vi "Create Plot Object.vi"(6 "Control Ref Queue":T1, 7 "Actual Transform In":T2, 8 "error in (no error)":errorcluster, 9 "Multiplot Representation In":T4, 10 "3D Bar.lvclass in":refnum<class "3D Bar.lvclass">, 11 "Plot Object In":refnum<vi>) -> (0 "error out":errorcluster, 1 "Multiplot Representation Out":T4, 2 "3D Bar.lvclass out":refnum<class "3D Bar.lvclass">, 3 "Plot Object Out":refnum<vi>, 5 "Actual Transform Out":T2)   [LabVIEW 2017, in "3D Bar.lvclass"]
uses:
  <vilib>/Math Plots/3D Math Plots/3D Bar/3D Bar/3D Bar.lvclass
  <vilib>/Math Plots/3D Math Plots/3D Plot/3D Plot/Typedef/Multiplot Representation.ctl
  <vilib>/Math Plots/3D Math Plots/3D Plot/3D Plot/Typedef/Plot Representation.ctl
  <vilib>/Math Plots/3D Math Plots/3D Plot/3D Plot/Typedef/Range Clusters.ctl
  <vilib>/Math Plots/3D Math Plots/3D Plot/3D Plot/Typedef/Mesh Data.ctl
  <vilib>/Math Plots/3D Math Plots/3D Plot/3D Plot/Typedef/Actual Transform.ctl
  <vilib>/Math Plots/3D Math Plots/3D Plot/Action String/3DMathPlot Ctrl Act Queue.ctl
  <vilib>/Math Plots/3D Math Plots/3D Plot/Action String/3DMathPlot Ctrl Act Cluster.ctl
  <vilib>/Math Plots/3D Math Plots/3D Plot/Action String/3DMathPlot State Class.ctl
  <vilib>/Math Plots/3D Math Plots/3D Bar/3D Bar/3D Bar.lvclass/3D Bar.ctl
  <vilib>/Math Plots/3D Math Plots/3D Plot/3D Plot/3D Plot.lvclass
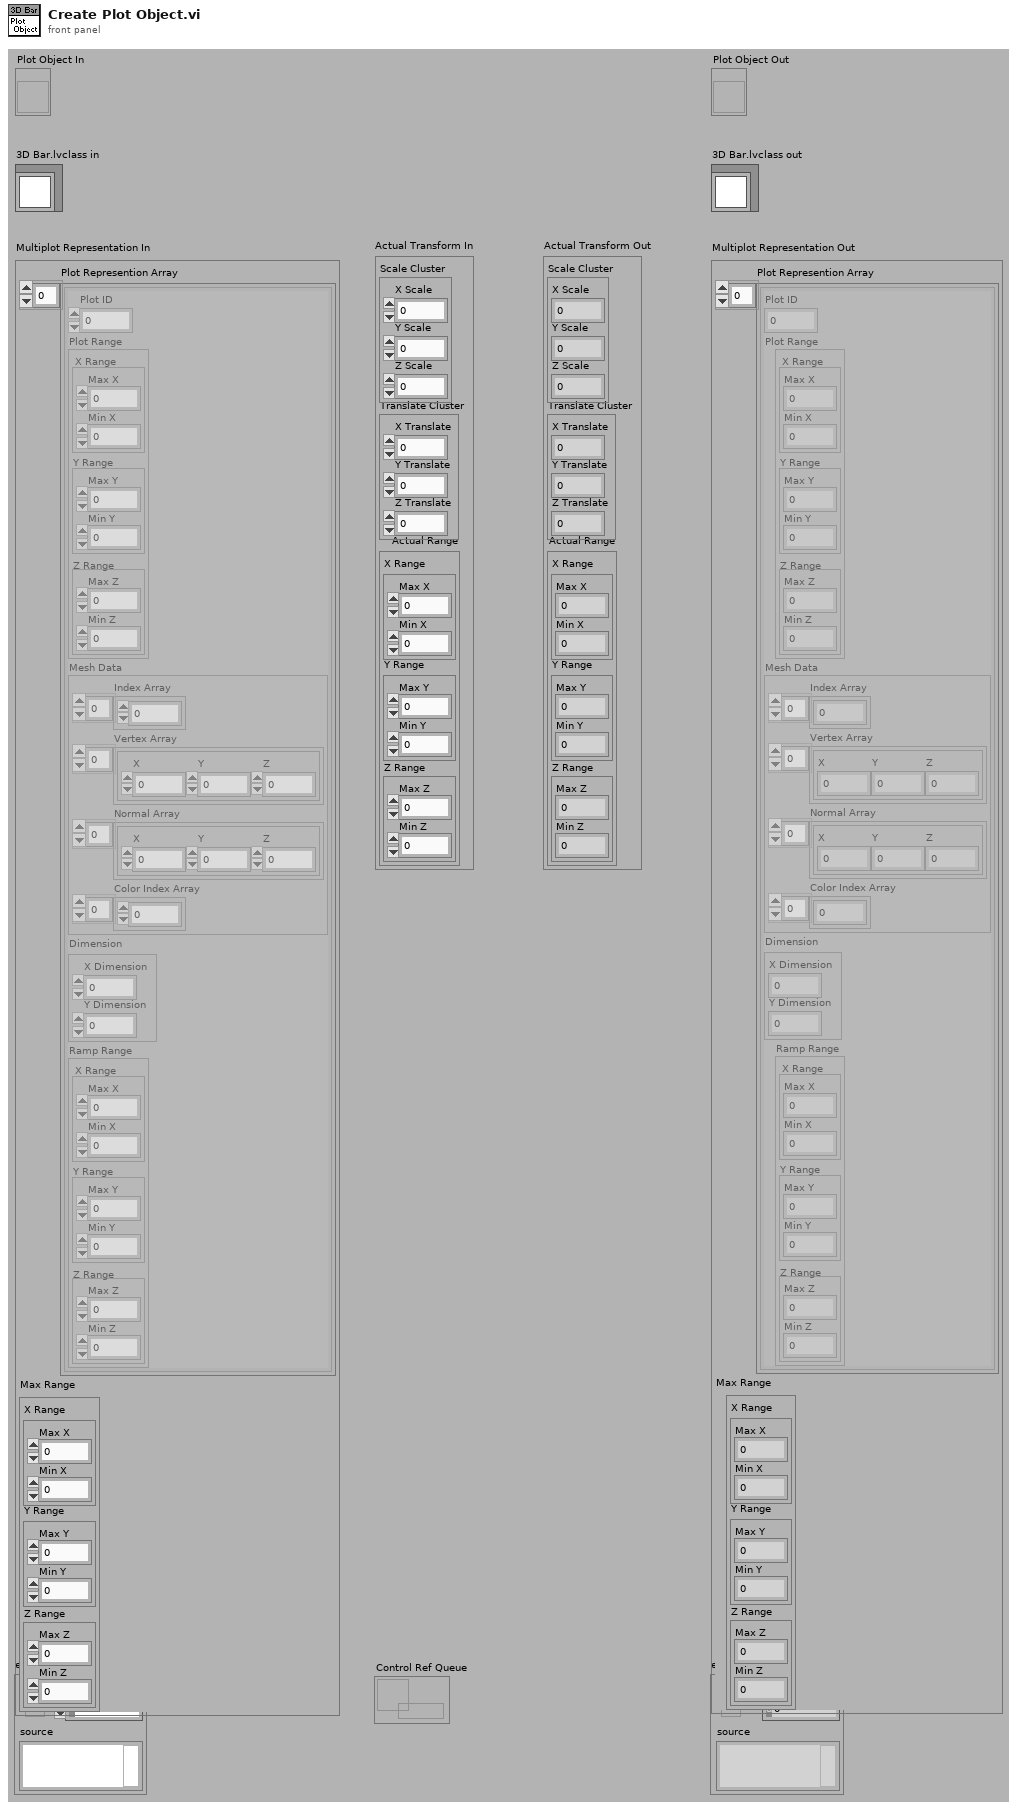
[diagram p1: front panel]
types:
  T1 = typedef "3DMathPlot Ctrl Act Queue.ctl" = refnum<queue>
  T2 = typedef "3D Plot.lvclass/Actual Transform.ctl" = cluster{"Scale Cluster":cluster{"X Scale":sgl, "Y Scale":sgl, "Z Scale":sgl}, "Translate Cluster":cluster{"X Translate":sgl, "Y Translate":sgl, "Z Translate":sgl}, "Actual Range":T3}
  T3 = typedef "3D Plot.lvclass/Range Clusters.ctl" = cluster{"X Range":cluster{"Max X":sgl, "Min X":sgl}, "Y Range":cluster{"Max Y":sgl, "Min Y":sgl}, "Z Range":cluster{"Max Z":sgl, "Min Z":sgl}}
  T4 = typedef "3D Plot.lvclass/Multiplot Representation.ctl" = cluster{"Plot Represention Array":T5[], "Max Range":T3}
  T5 = typedef "3D Plot.lvclass/Plot Representation.ctl" = cluster{"Plot ID":i32, "Plot Range":T3, "Mesh Data":T6, "Dimension":cluster{"X Dimension":i32, "Y Dimension":i32}, "Ramp Range":T3}
  T6 = typedef "3D Plot.lvclass/Mesh Data.ctl" = cluster{"Index Array":u32[], "Vertex Array":cluster{"X":sgl, "Y":sgl, "Z":sgl}[], "Normal Array":cluster{"X":sgl, "Y":sgl, "Z":sgl}[], "Color Index Array":i32[]}
  T7 = typedef "3D Bar.lvclass/3D Bar Property Array.ctl" = T8[]
  T8 = typedef "3D Bar.lvclass/3D Bar Property.ctl" = cluster{"General Property":cluster{"Plot Name":string, "Coordinate System":enum16{"Cartesian", "Cylindrical", "Spherical"}, "Opacity":sgl}, "Projection Property":cluster{"Draw XY":bool, "Draw YZ":bool, "Draw XZ":bool}, "Plot Property":cluster{"Line Style":T9, "Line Width":sgl, "Line Color":u32, "Antialiasing":bool}, "Bar Property":cluster{"Bar Mode":enum16{"Detach", "Group", "Stack"}, "Bar Width":sgl, "Color Pair Array":cluster{"Color":u32, "String":string}[]}}
  T9 = typedef "3D Plot.lvclass/Line Type.ctl" = enum16{"None", "Solid", "Dash", "Dot", "Dash Dot"}
  T10 = enum16{"Points", "Lines", "Line Strip", "Line Loop", "Triangles", "Triangle Strip", "Triangle Fan", "Quads", "Quad Strip", "Polygon"}
  T11 = cluster{"Draw XY":bool, "Draw YZ":bool, "Draw XZ":bool}
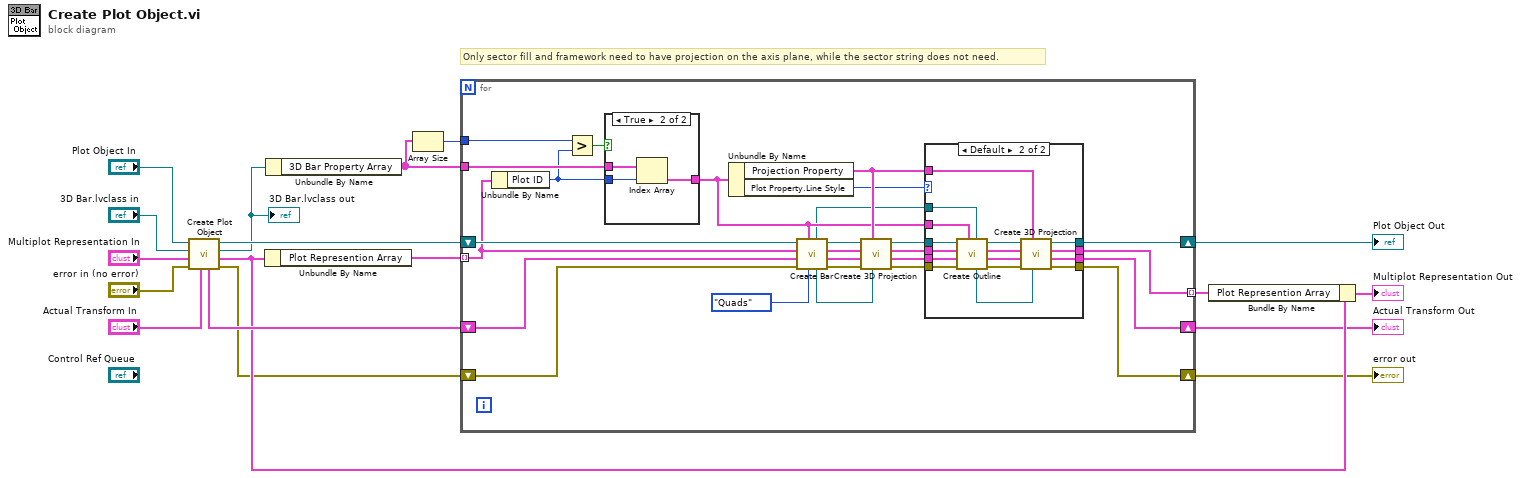
[diagram p0: block diagram]
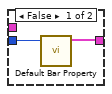
[diagram p2: hidden frame]
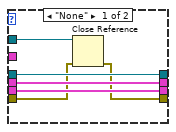
[diagram p3: hidden frame]
diagram:
  # "Only sector fill and framework need to have projection on the axis plane, while the sector string does not need."
  n1 = call-parent "Create Plot Object.vi"("Actual Transform In"="Actual Transform In", "error in (no error)"="error in (no error)", "Multiplot Representation In"="Multiplot Representation In", "3D Plot.lvclass in"="3D Bar.lvclass in", "Plot Object In"="Plot Object In") -> ("error out"=w3:errorcluster, "Multiplot Representation Out"=w10:T4, "3D Plot.lvclass out"=w4:refnum<class "3D Bar.lvclass">, "Plot Object Out"=w6:refnum<vi>, "Actual Transform Out"=w11:T2)  [unwired: 1 in, 1 out]
  "3D Bar.lvclass out" <- w4
  n2 = Unbundle By Name(w10) -> ("Plot Represention Array"=w18:T5[])
  n3 = Unbundle By Name(w4) -> ("3D Bar Property Array"=w1:T7)
  n4 = Array Size(array=w1) -> (size(s)=w2:i32)
  n5 = for {
    tunnel: [w38] -> w17 mode=indexing
    shift-right: [w37] -> w5
    shift-left: w6 -> [w41]
    shift-right: [w39] -> w7
    shift-left: w3 -> [w40]
    shift-right: [w36] -> w8
    shift-left: w11 -> [w42]
    tunnel: w18 -> [w28] mode=indexing
    tunnel: w1 -> [w25]
    tunnel: w2 -> [w22]
    n6 = Unbundle By Name(w28) -> ("Plot ID"=w24:i32)
    n7 = Greater?(x=w22, y=w24) -> (0:w26:bool)
    n8 = case shown="True" w26 {
      tunnel: w25 -> [_ w47]
      tunnel: [w43 w46] -> w23
      tunnel: w24 -> [w44 w45]
      frame False {
        n9 = call <vilib>:"Default Bar Property.vi"("Plot ID"=w44) -> ("Default Property"=w43:T8)  [unwired: 10 out]
      }
      frame True {
        n10 = Index Array(array=w47, index=w45) -> (element=w46:T8)
      }
    }
    n11 = Unbundle By Name(w23) -> ("Projection Property"=w29:T11, "Plot Property.Line Style"=w27:T9)
    n12 = call <vilib>:"Create Bar.vi"("Draw Mode"=T10."Quads", "3D Bar Property"=w23, "error in (no error)"=w40, "Plot Representation In"=w28, "Plot Object In"=w41) -> ("error out"=w35:errorcluster, "Plot Representation Out"=w32:T5, "Plot Object Out"=w34:refnum<vi>, "Sector Object Out"=w20:refnum<vi>, "Bar Drawable"=w19:refnum<vi>)  [unwired: 2 out]
    n13 = call <vilib>:"Create 3D Projection.vi"("Sub Object In"=w20, "Projection Property"=w29, "error in (no error)"=w35, "Actual Transform In"=w42, "Plot Object In"=w34) -> ("error out"=w33:errorcluster, "Actual Transform Out"=w30:T2, "Plot Object Out"=w31:refnum<vi>)  [unwired: 1 in, 3 out]
    n14 = case shown="Default" w27 {
      tunnel: [w48 w67] -> w39
      tunnel: [w52 w66] -> w38
      tunnel: [w53 w65] -> w37
      tunnel: [w51 w64] -> w36
      tunnel: w33 -> [w49 w63]
      tunnel: w32 -> [w52 w62]
      tunnel: w31 -> [w53 w61]
      tunnel: w30 -> [w51 w60]
      tunnel: w29 -> [_ w59]
      tunnel: w23 -> [_ w55]
      tunnel: w19 -> [w50 w54]
      frame "None" {
        n15 = Close Reference(reference=w50, error in (no error)=w49) -> (error out=w48:errorcluster)
      }
      frame Default {
        n16 = call <vilib>:"Create Outline.vi"("Bar Drawable"=w54, "3D Bar Property"=w55, "error in (no error)"=w63, "Plot Representation In"=w62, "Plot Object In"=w61) -> ("error out"=w57:errorcluster, "Plot Representation Out"=w66:T5, "Plot Object Out"=w56:refnum<vi>, "Sector Object Out"=w58:refnum<vi>)  [unwired: 3 out]
        n17 = call <vilib>:"Create 3D Projection.vi"("Sub Object In"=w58, "Projection Property"=w59, "error in (no error)"=w57, "Actual Transform In"=w60, "Plot Object In"=w56) -> ("error out"=w67:errorcluster, "Actual Transform Out"=w64:T2, "Plot Object Out"=w65:refnum<vi>)  [unwired: 1 in, 3 out]
      }
    }
  }
  "error out" <- w7
  "Plot Object Out" <- w5
  "Actual Transform Out" <- w8
  n18 = Bundle By Name(cluster=w10, "Plot Represention Array"=w17) -> (→"Multiplot Representation Out":T4)
